vi "Save Configuration.vi"(8 "error in (no error)":errorcluster, 11 "Configuration in":refnum<class "Configuration.lvclass">) -> (0 "error out":errorcluster, 2 "file path":path, 3 "Configuration out":refnum<class "Configuration.lvclass">)   [LabVIEW 2016, in "Configuration.lvlib" / "Configuration.lvclass"]
uses:
  Configuration.lvclass
  <vilib>/Utility/config.llb/NI_LVConfig.lvlib
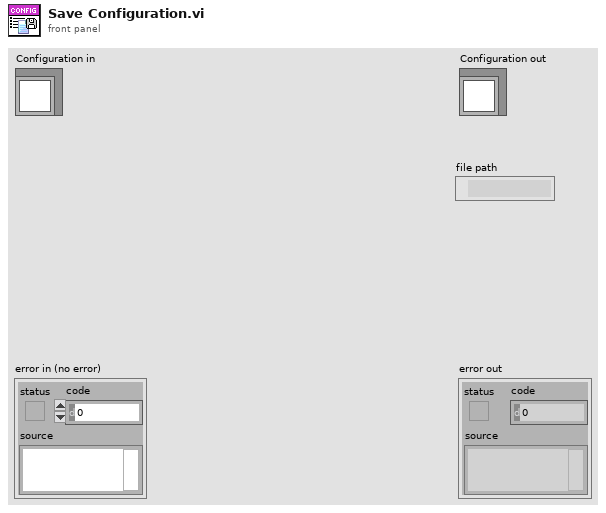
[diagram p1: front panel]
types:
  T1 = typedef "NI_LVConfig.lvlib/Config Data RefNum.ctl" = refnum<k1>
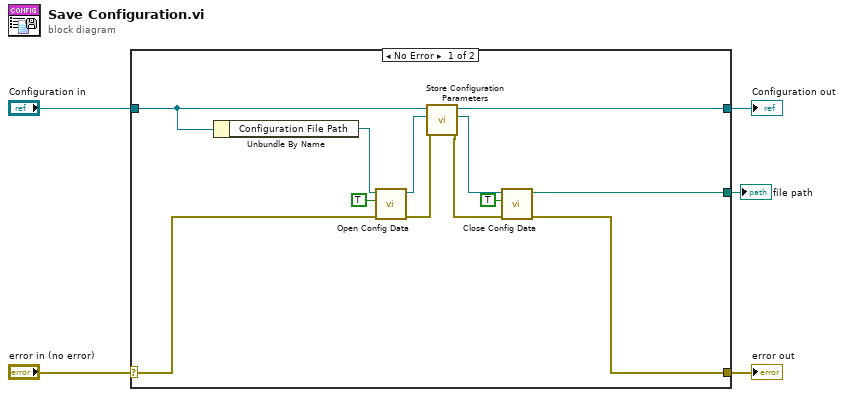
[diagram p0: block diagram]
diagram:
  n1 = case shown="No Error" "error in (no error)" {
    selector: "error in (no error)" -> [w14 w19]
    tunnel: [w13 w19] -> w4
    tunnel: [w7 w18] -> w2
    tunnel: "Configuration in" -> [w12 w18]
    tunnel: [w6 _] -> w1
    frame No Error {
      n2 = Unbundle By Name(w12) -> ("Configuration File Path"=w17:path)
      n3 = call <vilib>:"Open Config Data.vi"("error in (no error)"=w14, "create file if necessary (T)"=TRUE, "configuration file path"=w17) -> ("error out"=w10:errorcluster, "refnum"=w11:T1)  [unwired: 6 in, 1 out]
      n4 = call-dynamic "Store Configuration Parameters.vi"("error in (no error)"=w10, "refnum"=w11, "Configuration in"=w12) -> ("error out"=w9:errorcluster, "refnum out"=w8:T1, "Configuration out"=w7:refnum<class "Configuration.lvclass">)  [unwired: 6 in]
      n5 = call <vilib>:"Close Config Data.vi"("error in (no error)"=w9, "write file if changed (T)"=TRUE, "refnum"=w8) -> ("error out"=w13:errorcluster, "file path"=w6:path)  [unwired: 7 in]
    }
    frame Error {
    }
  }
  "error out" <- w4
  "Configuration out" <- w2
  "file path" <- w1
